vi "系统设置.vi"() -> ()   [LabVIEW 2016]
uses:
  <vilib>/Utility/miscctls.llb/LVPointTypeDef.ctl
  <vilib>/ptbypt/NI_PtbyPt.lvlib
  <vilib>/Utility/config.llb/NI_LVConfig.lvlib
  PLC/PLC.lvlib
panel:
  out "一级权限":bool
  in  "定时重启配置":bool
  in  "总磷":bool
  in  "模块启用配置":bool
  in  "短信报警设置":bool
  in  "首页显示设置":bool
  in  "跨度核查":bool
  in  "空白核查":bool
  out "选项卡控件":enum32{"自由设定", "国标协议", "流量设定"}(tab)
  in  "24H周期设置":bool[](xcontrol)
  in  "运行间隔":i16=4 min=1 max=24
  in  "流量阈值":dbl=4.0 min=1.0 max=24.0
  in  "时间阈值":u16=4 min=1 max=24
  in  "周期设置":enum16{"自由设定", "国标协议", "流量设定"}(ring)
  out "二级权限":bool
  in  "质控启动日期":string(combo)="关闭"
  in  "跨度核查时间":u16(ring)=6 items=["00H", "01H", "02H", "03H", "04H", "05H", "06H", "07H", "08H", "09H", "10H", "11H", "12H", "13H", "14H", "15H", "16H", "17H", "18H", "19H", "20H", "21H", "22H", "23H", "关闭"]
  in  "空白核查时间":u16(ring)=2 items=["00H", "01H", "02H", "03H", "04H", "05H", "06H", "07H", "08H", "09H", "10H", "11H", "12H", "13H", "14H", "15H", "16H", "17H", "18H", "19H", "20H", "21H", "22H", "23H", "关闭"]
  in  "CODCr":bool
  in  "总氮":bool
  in  "氨氮":bool
  in  "CODmn":bool
  in  "多参数":bool
  in  "输入密码":u32
  in  "布尔":bool
  in  "副屏显示设置":bool
  in  "开机启动":bool caption="氨氮禁用"
  in  "运行模式":enum16{"维护模式", "常规模式", "应急模式", "质控模式"}(ring)
  # "注：周期设置分为自由设定和国标协议两种。\n1：选择自由设定情况下：运行间隔将不可选用并变灰色，周期设置可自由手动勾选\n2：选择国标协议情况下：周期时间将由运行间隔选择的时间决定，下方周期设置被禁用并无法手动勾选。\n3：选择流量设定情况下：瞬时流量连续超过流量阈值到达时间阈值设定值，仪器将自动开启测量。"
  # "自动运行启动参数"
  # "质控频次："
  # "零点核查时间："
  # "跨度核查时间："
  # "启动周期设置"
  # "m3/S"
  # "秒"
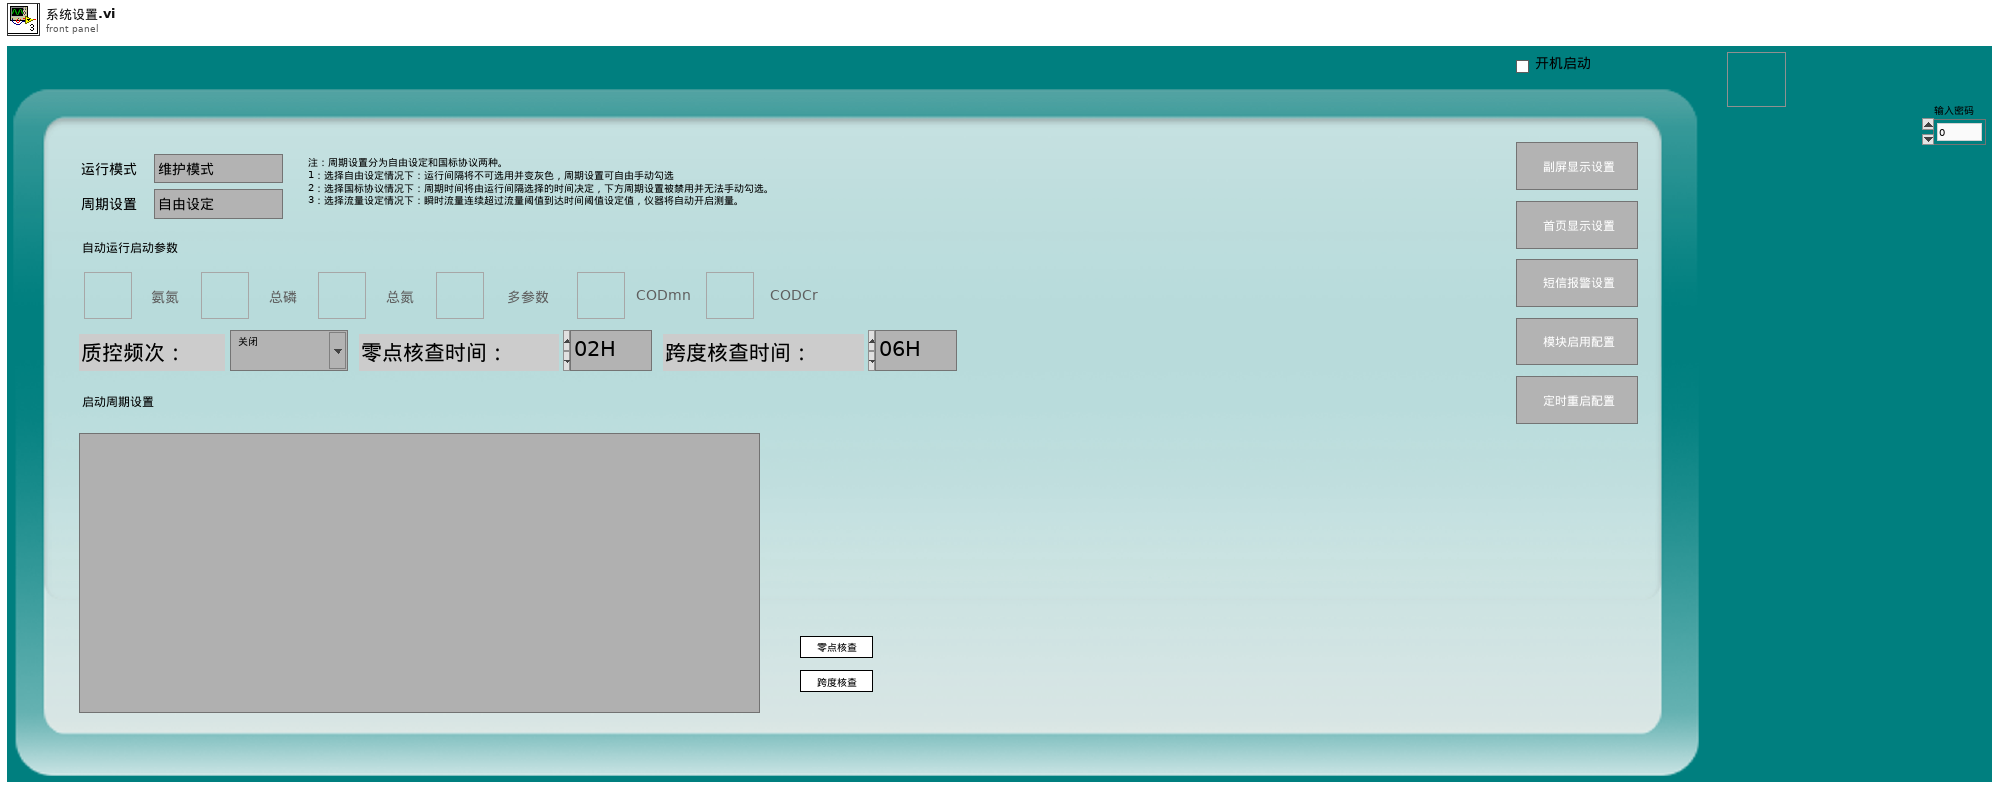
[diagram p1: front panel]
types:
  T1 = typedef "LVPointTypeDef.ctl" = cluster{"Horizontal":i16, "Vertical":i16}
  T2 = enum8{"Enabled", "Disabled", "Disabled and Grayed Out"}
  T3 = cluster{"频次":enum16{"关闭", "每天", "星期一", "星期二", "星期三", "星期四", "星期五", "星期六", "星期日"}, "时":u16, "分":u16}
  T4 = typedef "LVDateTimeRec.ctl" = cluster{"秒数的小数部分":dbl, "秒":i32, "分":i32, "时":i32, "日":i32, "月":i32, "年":i32, "天数（周）":i32, "天数（年）":i32, "DST":i32}
  T5 = enum16{"关闭", "每天", "星期一", "星期二", "星期三", "星期四", "星期五", "星期六", "星期日"}
  T6 = enum32{"Bad", "Idle", "Run top level", "Running"}
  T7 = typedef "NI_LVConfig.lvlib/Config Data RefNum.ctl" = refnum<k1>
  T8 = cluster{"运行模式":enum16{"维护模式", "常规模式", "应急模式", "质控模式"}}
  T9 = enum16{"启动测量", "标样核查", "零点核查", "跨度核查", "空白测试", "平行样测试", "加标回收", "空白校准", "标样校准", "初始化（清洗）", "停止测试", "仪器重启", "校时", "模式设置", "测量间隔设置"}
  T10 = cluster{"测量模式":enum16{"水样测量", "标样核查", "零点核查", "跨度核查", "空白测试", "加标回收", "平行样", "校零", "校标"}}
  T11 = cluster{"测试模式":enum16{"正常测试", "集成干预"}, "参数启用":cluster{"氨氮":bool, "总磷":bool, "总氮":bool, "多参数":bool, "CODMn":bool, "CODcr":bool}}
  T12 = cluster{"运行模式":enum16{"维护模式", "常规模式", "应急模式", "质控模式"}, "质控频次":enum16{"关闭", "每天", "星期一", "星期二", "星期三", "星期四", "星期五", "星期六", "星期日"}, "空白核查时间":u16, "跨度核查时间":u16, "24H周期设置":bool[]}
  T13 = enum32{"Invalid", "Standard", "Closed", "Hidden", "Minimized", "Maximized"}
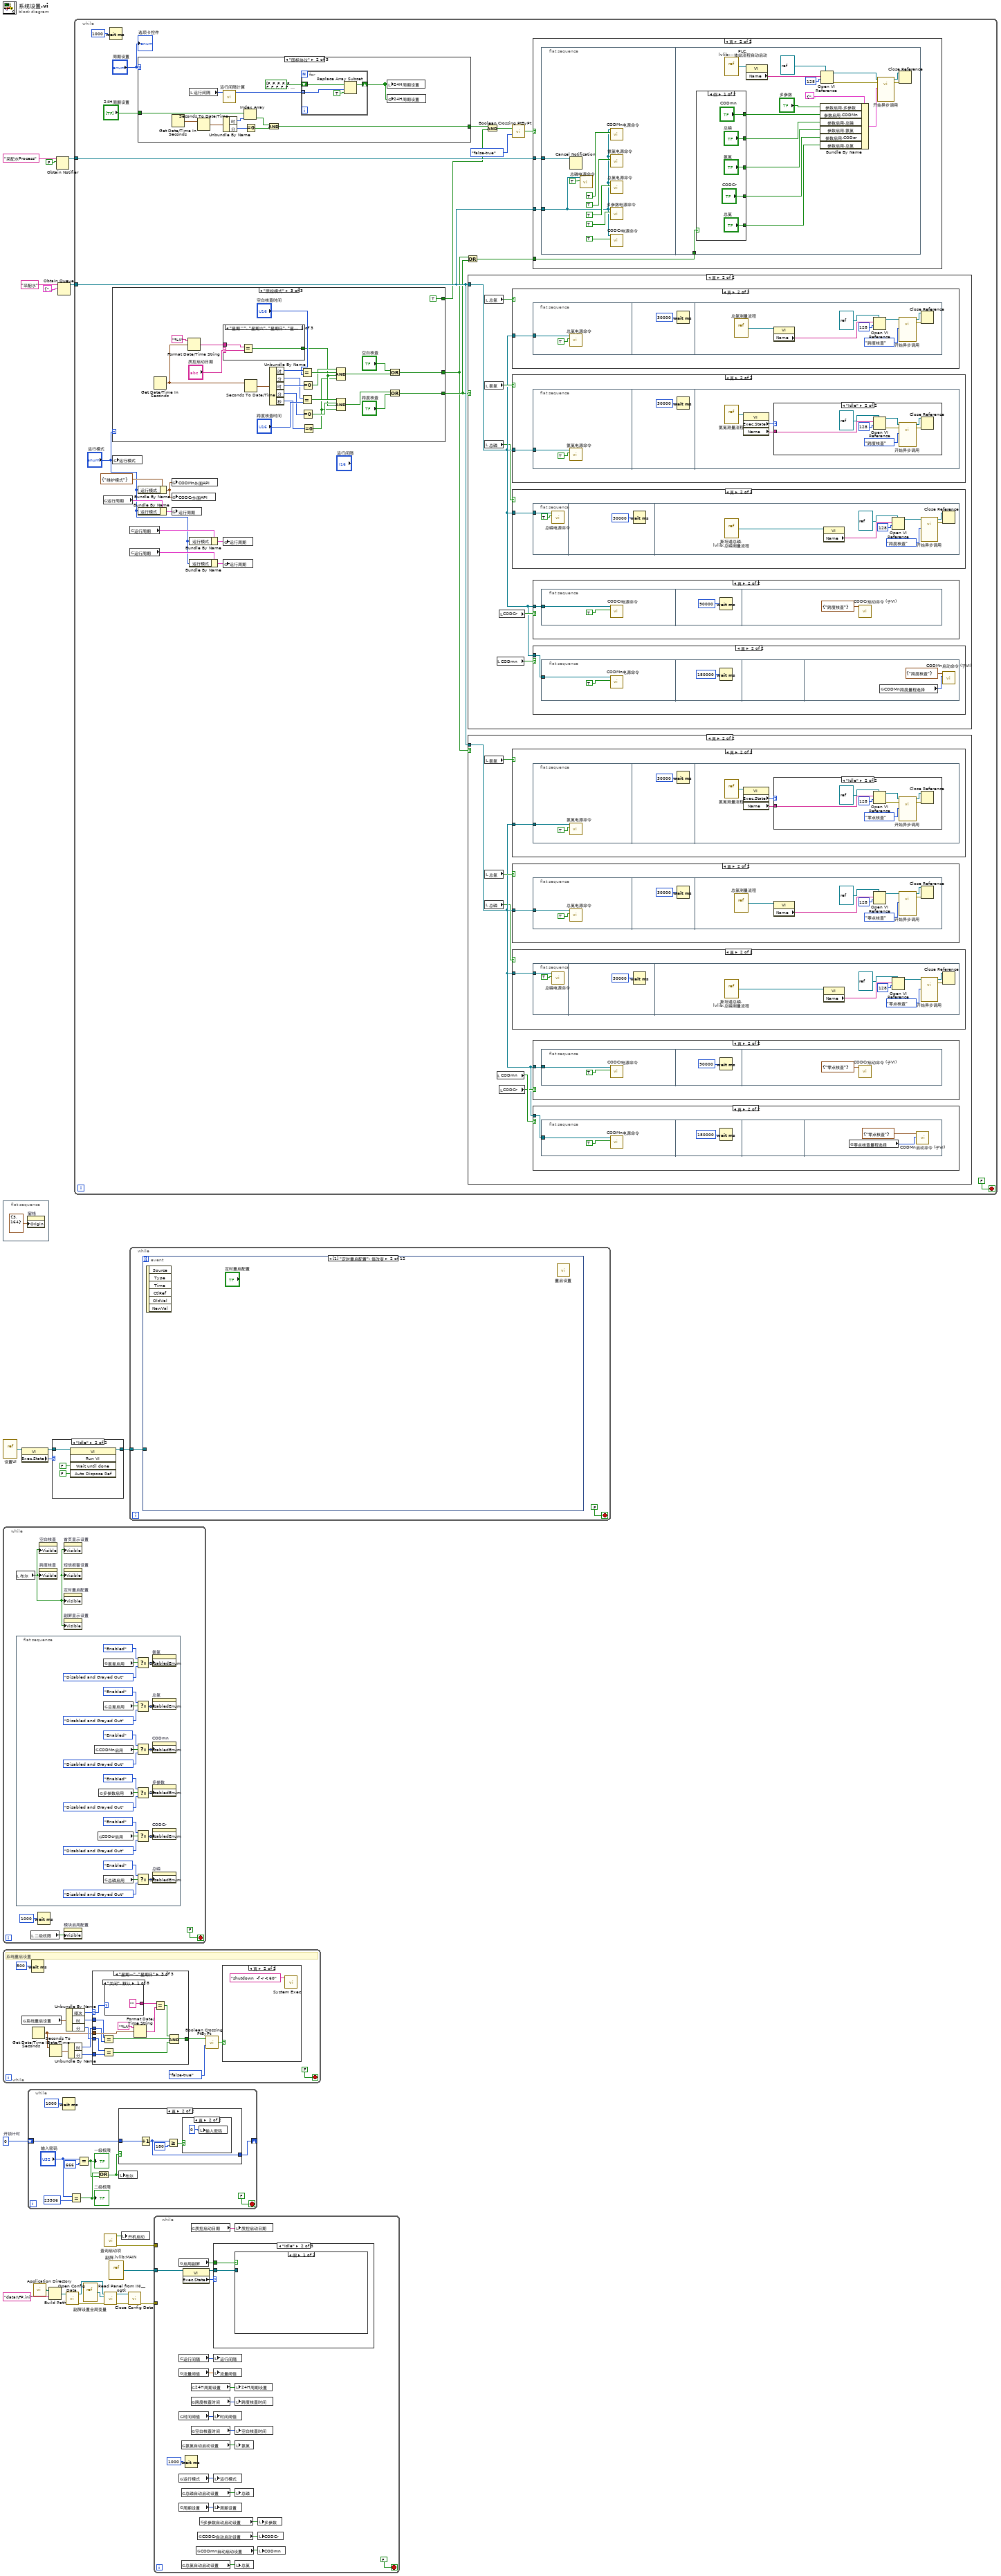
[diagram p0: block diagram]
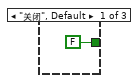
[diagram p3: hidden frame]
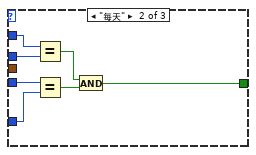
[diagram p4: hidden frame]
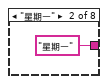
[diagram p5: hidden frame]
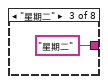
[diagram p6: hidden frame]
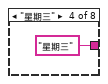
[diagram p7: hidden frame]
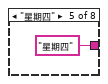
[diagram p8: hidden frame]
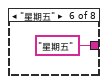
[diagram p9: hidden frame]
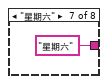
[diagram p10: hidden frame]
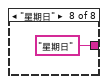
[diagram p11: hidden frame]
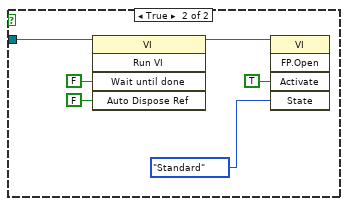
[diagram p16: hidden frame]
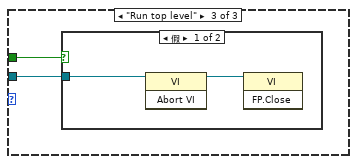
[diagram p17: hidden frame]
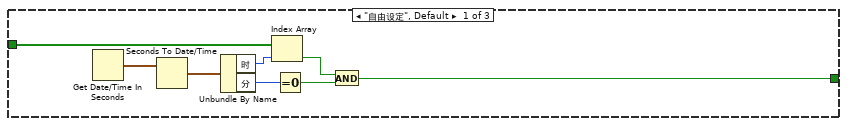
[diagram p19: hidden frame]
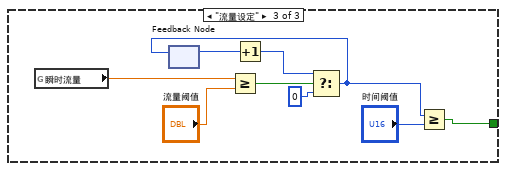
[diagram p20: hidden frame]
diagram:
  w19 = u32 0  # 开锁计时
  n1 = flat-sequence {
    frame #0 {
      n2 = property on="窗格" class="Pane"("Origin"=T1 {"Horizontal"=3, "Vertical"=164} ("原点")) -> ()  [unwired: 2 in, 2 out]
    }
  }
  n3 = vi-ref "设置UI.vi"() -> (w14:refnum<vi>)
  n4 = while {
    stop <- FALSE stop-if-true
    n5 = local read "布尔"() -> (w26:bool)
    n6 = flat-sequence {
      frame #0 {
        n7 = global read "系统设置全局变量.vi" "CODMn启用"() -> (w38:bool)
        n8 = global read "系统设置全局变量.vi" "CODcr启用"() -> (w39:bool)
        n9 = global read "系统设置全局变量.vi" "多参数启用"() -> (w37:bool)
        n10 = global read "系统设置全局变量.vi" "氨氮启用"() -> (w33:bool)
        n11 = global read "系统设置全局变量.vi" "总氮启用"() -> (w40:bool)
        n12 = global read "系统设置全局变量.vi" "总磷启用"() -> (w31:bool)
        n13 = Select(t=T2."Enabled" ("禁用"), s=w33, f=T2."Disabled and Grayed Out" ("禁用")) -> (s? t:f=w41:T2)
        n14 = Select(t=T2."Enabled" ("禁用"), s=w40, f=T2."Disabled and Grayed Out" ("禁用")) -> (s? t:f=w35:T2)
        n15 = Select(t=T2."Enabled" ("禁用"), s=w38, f=T2."Disabled and Grayed Out" ("禁用")) -> (s? t:f=w42:T2)
        n16 = Select(t=T2."Enabled" ("禁用"), s=w37, f=T2."Disabled and Grayed Out" ("禁用")) -> (s? t:f=w36:T2)
        n17 = Select(t=T2."Enabled" ("禁用"), s=w39, f=T2."Disabled and Grayed Out" ("禁用")) -> (s? t:f=w52:T2)
        n18 = Select(t=T2."Enabled" ("禁用"), s=w31, f=T2."Disabled and Grayed Out" ("禁用")) -> (s? t:f=w32:T2)
        n19 = property on="氨氮" class="Bool (严格)"("DisabledEnum"=w41) -> ()  [unwired: 2 in, 2 out]
        n20 = property on="总氮" class="Bool (严格)"("DisabledEnum"=w35) -> ()  [unwired: 2 in, 2 out]
        n21 = property on="CODmn" class="Bool (严格)"("DisabledEnum"=w42) -> ()  [unwired: 2 in, 2 out]
        n22 = property on="多参数" class="Bool (严格)"("DisabledEnum"=w36) -> ()  [unwired: 2 in, 2 out]
        n23 = property on="CODCr" class="Bool (严格)"("DisabledEnum"=w52) -> ()  [unwired: 2 in, 2 out]
        n24 = property on="总磷" class="Bool (严格)"("DisabledEnum"=w32) -> ()  [unwired: 2 in, 2 out]
      }
    }
    n25 = local read "二级权限"() -> (w25:bool)
    n26 = Wait (ms)(milliseconds to wait=u32 1000 ("等待时间（毫秒）")) -> ()  [unwired: 1 out]
    n27 = property on="空白核查" class="Bool"("Visible"=w26) -> ()  [unwired: 2 in, 2 out]
    n28 = property on="跨度核查" class="Bool"("Visible"=w26) -> ()  [unwired: 2 in, 2 out]
    n29 = property on="首页显示设置" class="Bool"("Visible"=w26) -> ()  [unwired: 2 in, 2 out]
    n30 = property on="短信报警设置" class="Bool"("Visible"=w26) -> ()  [unwired: 2 in, 2 out]
    n31 = property on="定时重启配置" class="Bool"("Visible"=w26) -> ()  [unwired: 2 in, 2 out]
    n32 = property on="副屏显示设置" class="Bool"("Visible"=w26) -> ()  [unwired: 2 in, 2 out]
    n33 = property on="模块启用配置" class="Bool"("Visible"=w25) -> ()  [unwired: 2 in, 2 out]
  }
  n34 = while {
    stop <- FALSE stop-if-true
    # "系统重启设置"
    n35 = global read "系统设置全局变量.vi" "系统重启设置"() -> (w65:T3)
    n36 = Wait (ms)(milliseconds to wait=u32 500 ("等待时间（毫秒）")) -> ()  [unwired: 1 out]
    n37 = Get Date/Time In Seconds() -> (seconds since 1Jan1904=w56:timestamp)
    n38 = Seconds To Date/Time(time stamp (now)=w56) -> (date time rec=w63:T4)  [unwired: 1 in]
    n39 = Unbundle By Name(w65) -> ("频次"=w64:T5, "时"=w60:u16, "分"=w59:u16)
    n40 = Unbundle By Name(w63) -> ("时"=w62:i32, "分"=w61:i32)
    n41 = case shown="\"星期一\"..\"星期日\"" w64 {
      selector: w64 -> [_ _ w85]
      tunnel: [FALSE w68 w75] -> w55
      tunnel: w62 -> [_ w74 w79]
      tunnel: w61 -> [_ w71 w77]
      tunnel: w60 -> [_ w73 w80]
      tunnel: w59 -> [_ w72 w78]
      tunnel: w56 -> [_ _ w86]
      frame "关闭", Default {
      }
      frame "每天" {
        n42 = Equal?(x=w73, y=w74) -> (x = y?=w69:bool)
        n43 = Equal?(x=w72, y=w71) -> (x = y?=w70:bool)
        n44 = And(x=w69, y=w70) -> (x .and. y?=w68:bool)
      }
      frame "星期一".."星期日" {
        n45 = Equal?(x=w80, y=w79) -> (x = y?=w81:bool)
        n46 = Equal?(x=w78, y=w77) -> (x = y?=w82:bool)
        n47 = case shown="\"关闭\", 默认" w85 {
          tunnel: ["" ("时间格式字符串(%c)") "星期一" ("时间格式字符串(%c)") "星期二" ("时间格式字符串(%c)") "星期三" ("时间格式字符串(%c)") "星期四" ("时间格式字符串(%c)") "星期五" ("时间格式字符串(%c)") "星期六" ("时间格式字符串(%c)") "星期日" ("时间格式字符串(%c)")] -> w83
          frame "关闭", Default {
          }
          frame "星期一" {
          }
          frame "星期二" {
          }
          frame "星期三" {
          }
          frame "星期四" {
          }
          frame "星期五" {
          }
          frame "星期六" {
          }
          frame "星期日" {
          }
        }
        n48 = Format Date/Time String(time format string (%c)="%A" ("时间格式字符串(%c)"), seconds (now)=w86) -> (date/time string=w84:string)  [unwired: 1 in]
        n49 = Equal?(x=w83, y=w84) -> (x = y?=w76:bool)
        n50 = Compound Arithmetic op=AND ("复合运算")(w76, w81, w82) -> (w75:bool)
      }
    }
    n51 = call <vilib>:"Boolean Crossing PtByPt.vi"("direction"=enum16{"either", "false-true", "true-false"}."false-true", "input"=w55) -> ("crossing"=w53:bool)  [unwired: 1 in]
    n52 = case shown="真" w53 {
      frame False {
      }
      frame True {
        n53 = call <vilib>:"System Exec.vi"("command line"="shutdown  -f -r -t 60") -> ()  [unwired: 7 in, 4 out]
      }
    }
  }
  n54 = property class="VI"(reference=w14) -> (reference out=w12:refnum<vi>, "Exec.State"=w13:T6)  [unwired: 1 in, 1 out]
  n55 = while {
    shift-right: [w101] -> _
    shift-left: w19 -> [w102]
    stop <- FALSE stop-if-true
    n56 = Wait (ms)(milliseconds to wait=u32 1000 ("等待时间（毫秒）")) -> ()  [unwired: 1 out]
    n57 = Equal?(x="输入密码", y=u32 23506) -> (x = y?=w98:bool)
    "二级权限" <- w98
    n58 = Equal?(x="输入密码", y=u32 666) -> (x = y?=w97:bool)
    "一级权限" <- w97
    n59 = Or(x=w98, y=w97) -> (x .or. y?=w96:bool)
    n60 = case shown="真" w96 {
      tunnel: w102 -> [_ w109]
      tunnel: [_ w108] -> w101
      frame False {
      }
      frame True {
        n61 = Increment(x=w109) -> (x+1=w108:u32)
        n62 = Greater Or Equal?(x=w108, y=u32 180) -> (x >= y?=w106:bool)
        n63 = case shown="真" w106 {
          frame False {
          }
          frame True {
            n64 = local write "输入密码"(u32 0 ("输入密码")) -> ()
          }
        }
      }
    }
    n65 = local write "布尔"(w96) -> ()
  }
  n66 = call <vilib>:"Application Directory.vi"() -> ("Application Directory"=w1:path)
  n67 = Build Path(base path=w1, name or relative path="data\\FP.ini" ("名称或相对路径")) -> (appended path=w8:path)
  n68 = case shown="\"Idle\"" w13 {
    tunnel: w12 -> [w111 w115]
    tunnel: [w111 w114] -> w11
    frame "Bad", Default {
    }
    frame "Idle" {
      n69 = invoke class="VI" method="Run VI"(reference=w115, "Wait until done"=FALSE ("结束前等待"), "Auto Dispose Ref"=FALSE ("自动销毁引用")) -> (reference out=w114:refnum<vi>)  [unwired: 2 in, 4 out]
    }
  }
  n70 = Obtain Notifier(name (unnamed)="采配水Process" ("名称（未命名）"), notification data type=FALSE) -> (notifier out=w21:refnum<notifier>)  [unwired: 2 in, 2 out]
  n71 = Obtain Queue(name (unnamed)="采配水" ("名称（未命名）"), element data type=cluster{"命令":string, "数据":variant} {"命令"="", "数据"=variant}) -> (queue out=w16:refnum<queue>)  [unwired: 3 in, 2 out]
  n72 = call <vilib>:"Open Config Data.vi"("configuration file path"=w8) -> ("error out"=w7:errorcluster, "refnum"=w4:T7)  [unwired: 8 in, 1 out]
  n73 = while {
    tunnel: w21 -> [w136]
    tunnel: w16 -> [w132]
    stop <- FALSE stop-if-true
    n74 = global read "氨氮断电保存全局变量.vi" "运行周期"() -> (w122:T12)
    n75 = Wait (ms)(milliseconds to wait=u32 1000 ("等待时间（毫秒）")) -> ()  [unwired: 1 out]
    n76 = case shown="\"质控模式\"" "运行模式" {
      tunnel: [_ _ w318] -> w125
      tunnel: [_ _ w322] -> w124
      tunnel: [_ TRUE TRUE] -> w129
      frame "维护模式", Default {
      }
      frame "常规模式" {
      }
      frame "质控模式" {
        n77 = Get Date/Time In Seconds() -> (seconds since 1Jan1904=w329:timestamp)
        n78 = Format Date/Time String(time format string (%c)="%A" ("时间格式字符串(%c)"), seconds (now)=w329) -> (date/time string=w327:string)  [unwired: 1 in]
        n79 = case shown="\"星期二\", \"星期六\", \"星期日\", \"星期三\", \"星期四\", \"星期五\", \"星期一\"" "质控启动日期" {
          selector: "质控启动日期" -> [w345 _ _]
          tunnel: [w344 TRUE FALSE] -> w330
          tunnel: w327 -> [w343 _ _]
          frame "星期二", "星期六", "星期日", "星期三", "星期四", "星期五", "星期一" {
            n80 = Equal?(x=w343, y=w345) -> (x = y?=w344:bool)
          }
          frame "每天" {
          }
          frame "关闭", Default {
          }
        }
        n81 = Seconds To Date/Time(time stamp (now)=w329) -> (date time rec=w342:T4)  [unwired: 1 in]
        n82 = Unbundle By Name(w342) -> ("时"=w341:i32, "分"=w339:i32, "时"=w335:i32, "分"=w334:i32, "秒"=w326:i32)
        n83 = Equal?(x=w341, y="空白核查时间") -> (x = y?=w338:bool)
        n84 = Equal?(x=w335, y="跨度核查时间") -> (x = y?=w333:bool)
        n85 = Equal To 0?(x=w339) -> (x = 0?=w337:bool)
        n86 = Equal To 0?(x=w334) -> (x = 0?=w332:bool)
        n87 = Equal To 0?(x=w326) -> (x = 0?=w325:bool)
        n88 = Compound Arithmetic op=AND ("复合运算")(w337, w338, w330, w325) -> (w323:bool)
        n89 = Compound Arithmetic op=AND ("复合运算")(w333, w332, w330, w325) -> (w320:bool)
        n90 = Or(x="空白核查", y=w323) -> (x .or. y?=w322:bool)
        n91 = Or(x=w320, y="跨度核查") -> (x .or. y?=w318:bool)
      }
    }
    n92 = global write "多参数全局变量.vi" "运行模式"("运行模式") -> ()
    n93 = global read "总氮断电保存全局变量.vi" "运行周期"() -> (w120:T12)
    n94 = global read "总磷断电保存全局变量.vi" "运行周期"() -> (w118:T12)
    n95 = case shown="\"国标协议\"" "周期设置" {
      tunnel: [w140 w147 w163] -> w128
      tunnel: "24H周期设置" -> [w139 w148 _]
      frame "自由设定", Default {
        n96 = Get Date/Time In Seconds() -> (seconds since 1Jan1904=w141:timestamp)
        n97 = Seconds To Date/Time(time stamp (now)=w141) -> (date time rec=w142:T4)  [unwired: 1 in]
        n98 = Unbundle By Name(w142) -> ("时"=w145:i32, "分"=w143:i32)
        n99 = Index Array(array=w139, index=w145) -> (element=w146:bool)
        n100 = Equal To 0?(x=w143) -> (x = 0?=w144:bool)
        n101 = And(x=w146, y=w144) -> (x .and. y?=w140:bool)
      }
      frame "国标协议" {
        n102 = Get Date/Time In Seconds() -> (seconds since 1Jan1904=w149:timestamp)
        n103 = local read "运行间隔"() -> (w158:i16)
        n104 = Seconds To Date/Time(time stamp (now)=w149) -> (date time rec=w150:T4)  [unwired: 1 in]
        n105 = call "运行间隔计算.vi"("运行周期"=w158) -> ("数组"=w157:i32[])  [unwired: 10 in]
        n106 = Unbundle By Name(w150) -> ("时"=w153:i32, "分"=w151:i32)
        n107 = Index Array(array=w148, index=w153) -> (element=w154:bool)
        n108 = Equal To 0?(x=w151) -> (x = 0?=w152:bool)
        n109 = And(x=w154, y=w152) -> (x .and. y?=w147:bool)
        n110 = for {
          tunnel: w157 -> [w161] mode=indexing
          shift-right: [w159] -> w155
          shift-left: bool[] [FALSE, FALSE, FALSE, FALSE, FALSE, FALSE, FALSE, FALSE, FALSE, FALSE, FALSE, FALSE, FALSE, FALSE, FALSE, FALSE, FALSE, FALSE, FALSE, FALSE, FALSE, FALSE, FALSE, FALSE] ("24H周期设置") -> [w162]
          n111 = Replace Array Subset(array=w162, new element=TRUE ("新元素/子数组"), index=w161) -> (w159:bool[])
        }
        n112 = local write "24H周期设置"(w155) -> ()
        n113 = global write "系统设置全局变量.vi" "24H周期设置"(w155) -> ()
      }
      frame "流量设定" {
        n114 = global read "流量计全局变量.vi" "瞬时流量"() -> (w171:dbl)
        n115 = feedback #1() -> (w168:i16)  [unwired: 1 in]
        n116 = Greater Or Equal?(x=w171, y="流量阈值") -> (x >= y?=w166:bool)
        n117 = Increment(x=w168) -> (x+1=w167:i16)
        n118 = Select(t=w167, s=w166, f=i16 0) -> (s? t:f=w165:i16)
        n119 = feedback-in #1(w165) -> ()
        n120 = Greater Or Equal?(x=w165, y="时间阈值") -> (x >= y?=w163:bool)
      }
    }
    n121 = Bundle By Name(cluster=T8 {"运行模式"=enum."维护模式"} ("外围API"), "运行模式"="运行模式") -> (w126:T8)
    n122 = Bundle By Name(cluster=w122, "运行模式"="运行模式") -> (w121:T12)
    n123 = global write "CODMN外部API.vi" "CODMn外围API"(w126) -> ()
    n124 = global write "CODCr外部API.vi" "CODCr外围API"(w126) -> ()
    n125 = global write "氨氮断电保存全局变量.vi" "运行周期"(w121) -> ()
    n126 = Bundle By Name(cluster=w120, "运行模式"="运行模式") -> (w119:T12)
    n127 = Bundle By Name(cluster=w118, "运行模式"="运行模式") -> (w117:T12)
    n128 = global write "总氮断电保存全局变量.vi" "运行周期"(w119) -> ()
    n129 = global write "总磷断电保存全局变量.vi" "运行周期"(w117) -> ()
    n130 = Or(x=w124, y=w125) -> (x .or. y?=w123:bool)
    n131 = case shown="真" w125 {
      tunnel: w132 -> [_ w173]
      frame False {
      }
      frame True {
        n132 = local read "总氮"() -> (w176:bool)
        n133 = local read "氨氮"() -> (w177:bool)
        n134 = local read "总磷"() -> (w172:bool)
        n135 = local read "CODmn"() -> (w175:bool)
        n136 = local read "CODCr"() -> (w174:bool)
        n137 = case shown="真" w176 {
          tunnel: w173 -> [_ w201]
          frame False {
          }
          frame True {
            n138 = flat-sequence {
              tunnel: w201 -> [w203]
              frame #0 {
                n139 = call "总氮电源命令.vi"("通电/断电"=TRUE, "队列"=w203) -> ()  [unwired: 9 in, 1 out]
              }
              frame #1 {
                n140 = Wait (ms)(milliseconds to wait=u32 30000 ("等待时间（毫秒）")) -> ()  [unwired: 1 out]
              }
              frame #2 {
                n141 = vi-ref "总氮测量流程.vi"() -> (w210:refnum<vi>)
                n142 = property class="VI"(reference=w210) -> ("Name"=w211:string)  [unwired: 1 in, 2 out]
                n143 = Open VI Reference(type specifier VI Refnum (for type only)=refnum<vi> refnum, vi path=w211, options=128 ("选项")) -> (vi reference=w209:refnum<vi>)  [unwired: 3 in, 1 out]
                n144 = call-by-ref "开始异步调用"(reference=w209, "控制命令"=T9."跨度核查") -> (reference out=w208:refnum<vi>, error out=w207:errorcluster)  [unwired: 12 in]
                n145 = Close Reference(reference=w208, error in (no error)=w207) -> ()  [unwired: 1 out]
              }
            }
          }
        }
        n146 = case shown="真" w177 {
          tunnel: w173 -> [_ w213]
          frame False {
          }
          frame True {
            n147 = flat-sequence {
              tunnel: w213 -> [w214]
              frame #0 {
                n148 = call "氨氮电源命令.vi"("通电/断电"=TRUE, "队列"=w214) -> ()  [unwired: 9 in, 1 out]
              }
              frame #1 {
                n149 = Wait (ms)(milliseconds to wait=u32 30000 ("等待时间（毫秒）")) -> ()  [unwired: 1 out]
              }
              frame #2 {
                n150 = vi-ref "氨氮测量流程.vi"() -> (w219:refnum<vi>)
                n151 = property class="VI"(reference=w219) -> ("Exec.State"=w217:T6, "Name"=w218:string)  [unwired: 1 in, 2 out]
                n152 = case shown="\"Idle\"" w217 {
                  tunnel: w218 -> [_ w224]
                  frame "Bad", Default {
                  }
                  frame "Idle" {
                    n153 = Open VI Reference(type specifier VI Refnum (for type only)=refnum<vi> refnum, vi path=w224, options=128 ("选项")) -> (vi reference=w222:refnum<vi>, error out=w225:errorcluster)  [unwired: 3 in]
                    n154 = call-by-ref "开始异步调用"(reference=w222, error in=w225, "控制命令"=T9."跨度核查") -> (reference out=w226:refnum<vi>, error out=w227:errorcluster)  [unwired: 11 in]
                    n155 = Close Reference(reference=w226, error in (no error)=w227) -> ()  [unwired: 1 out]
                  }
                }
              }
            }
          }
        }
        n156 = case shown="真" w172 {
          tunnel: w173 -> [_ w178]
          frame False {
          }
          frame True {
            n157 = flat-sequence {
              tunnel: w178 -> [w180]
              frame #0 {
                n158 = call "总磷电源命令.vi"("通电/断电"=TRUE, "队列"=w180) -> ()  [unwired: 9 in, 1 out]
              }
              frame #1 {
                n159 = Wait (ms)(milliseconds to wait=u32 30000 ("等待时间（毫秒）")) -> ()  [unwired: 1 out]
              }
              frame #2 {
                n160 = vi-ref "斯坦道总磷.lvlib:总磷测量流程.vi"() -> (w187:refnum<vi>)
                n161 = property class="VI"(reference=w187) -> ("Name"=w188:string)  [unwired: 1 in, 2 out]
                n162 = Open VI Reference(type specifier VI Refnum (for type only)=refnum<vi> refnum, vi path=w188, options=128 ("选项")) -> (vi reference=w186:refnum<vi>)  [unwired: 3 in, 1 out]
                n163 = call-by-ref "开始异步调用"(reference=w186, "控制命令"=T9."跨度核查") -> (reference out=w185:refnum<vi>, error out=w184:errorcluster)  [unwired: 12 in]
                n164 = Close Reference(reference=w185, error in (no error)=w184) -> ()  [unwired: 1 out]
              }
            }
          }
        }
        n165 = case shown="真" w174 {
          tunnel: w173 -> [_ w190]
          frame False {
          }
          frame True {
            n166 = flat-sequence {
              tunnel: w190 -> [w191]
              frame #0 {
                n167 = call "CODCr电源命令.vi"("通电/断电"=TRUE, "队列"=w191) -> ()  [unwired: 9 in, 1 out]
              }
              frame #1 {
                n168 = Wait (ms)(milliseconds to wait=u32 90000 ("等待时间（毫秒）")) -> ()  [unwired: 1 out]
              }
              frame #2 {
                n169 = call "CODCr启动命令 (子VI).vi"("启动测量模式"=T10 {"测量模式"=enum."跨度核查"}) -> ()  [unwired: 11 in]
              }
            }
          }
        }
        n170 = case shown="真" w175 {
          tunnel: w173 -> [_ w195]
          frame False {
          }
          frame True {
            n171 = flat-sequence {
              tunnel: w195 -> [w196]
              frame #0 {
                n172 = call "CODMn电源命令.vi"("通电/断电"=TRUE, "队列"=w196) -> ()  [unwired: 9 in, 1 out]
              }
              frame #1 {
                n173 = Wait (ms)(milliseconds to wait=u32 180000 ("等待时间（毫秒）")) -> ()  [unwired: 1 out]
              }
              frame #2 {
              }
              frame #3 {
                n174 = global read "CODMn断电保存全局变量.vi" "CODMn跨度量程选择"() -> (w199:enum32{"H", "L", "AUTO"})
                n175 = call "CODMn启动命令 (子VI).vi"("CODMn量程切换"=w199, "启动测量模式"=T10 {"测量模式"=enum."跨度核查"}) -> ()  [unwired: 10 in]
              }
            }
          }
        }
      }
    }
    n176 = case shown="真" w124 {
      tunnel: w132 -> [_ w229]
      frame False {
      }
      frame True {
        n177 = local read "氨氮"() -> (w233:bool)
        n178 = local read "总氮"() -> (w232:bool)
        n179 = local read "总磷"() -> (w228:bool)
        n180 = local read "CODmn"() -> (w231:bool)
        n181 = local read "CODCr"() -> (w230:bool)
        n182 = case shown="真" w233 {
          tunnel: w229 -> [_ w269]
          frame False {
          }
          frame True {
            n183 = flat-sequence {
              tunnel: w269 -> [w270]
              frame #0 {
                n184 = call "氨氮电源命令.vi"("通电/断电"=TRUE, "队列"=w270) -> ()  [unwired: 9 in, 1 out]
              }
              frame #1 {
                n185 = Wait (ms)(milliseconds to wait=u32 30000 ("等待时间（毫秒）")) -> ()  [unwired: 1 out]
              }
              frame #2 {
                n186 = vi-ref "氨氮测量流程.vi"() -> (w275:refnum<vi>)
                n187 = property class="VI"(reference=w275) -> ("Exec.State"=w273:T6, "Name"=w274:string)  [unwired: 1 in, 2 out]
                n188 = case shown="\"Idle\"" w273 {
                  tunnel: w274 -> [_ w280]
                  frame "Bad", Default {
                  }
                  frame "Idle" {
                    n189 = Open VI Reference(type specifier VI Refnum (for type only)=refnum<vi> refnum, vi path=w280, options=128 ("选项")) -> (vi reference=w278:refnum<vi>, error out=w281:errorcluster)  [unwired: 3 in]
                    n190 = call-by-ref "开始异步调用"(reference=w278, error in=w281, "控制命令"=T9."零点核查") -> (reference out=w282:refnum<vi>, error out=w283:errorcluster)  [unwired: 11 in]
                    n191 = Close Reference(reference=w282, error in (no error)=w283) -> ()  [unwired: 1 out]
                  }
                }
              }
            }
          }
        }
        n192 = case shown="真" w232 {
          tunnel: w229 -> [_ w257]
          frame False {
          }
          frame True {
            n193 = flat-sequence {
              tunnel: w257 -> [w259]
              frame #0 {
                n194 = call "总氮电源命令.vi"("通电/断电"=TRUE, "队列"=w259) -> ()  [unwired: 9 in, 1 out]
              }
              frame #1 {
                n195 = Wait (ms)(milliseconds to wait=u32 30000 ("等待时间（毫秒）")) -> ()  [unwired: 1 out]
              }
              frame #2 {
                n196 = vi-ref "总氮测量流程.vi"() -> (w266:refnum<vi>)
                n197 = property class="VI"(reference=w266) -> ("Name"=w267:string)  [unwired: 1 in, 2 out]
                n198 = Open VI Reference(type specifier VI Refnum (for type only)=refnum<vi> refnum, vi path=w267, options=128 ("选项")) -> (vi reference=w265:refnum<vi>)  [unwired: 3 in, 1 out]
                n199 = call-by-ref "开始异步调用"(reference=w265, "控制命令"=T9."零点核查") -> (reference out=w264:refnum<vi>, error out=w263:errorcluster)  [unwired: 12 in]
                n200 = Close Reference(reference=w264, error in (no error)=w263) -> ()  [unwired: 1 out]
              }
            }
          }
        }
        n201 = case shown="真" w228 {
          tunnel: w229 -> [_ w234]
          frame False {
          }
          frame True {
            n202 = flat-sequence {
              tunnel: w234 -> [w236]
              frame #0 {
                n203 = call "总磷电源命令.vi"("通电/断电"=TRUE, "队列"=w236) -> ()  [unwired: 9 in, 1 out]
              }
              frame #1 {
                n204 = Wait (ms)(milliseconds to wait=u32 30000 ("等待时间（毫秒）")) -> ()  [unwired: 1 out]
              }
              frame #2 {
                n205 = vi-ref "斯坦道总磷.lvlib:总磷测量流程.vi"() -> (w243:refnum<vi>)
                n206 = property class="VI"(reference=w243) -> ("Name"=w244:string)  [unwired: 1 in, 2 out]
                n207 = Open VI Reference(type specifier VI Refnum (for type only)=refnum<vi> refnum, vi path=w244, options=128 ("选项")) -> (vi reference=w242:refnum<vi>)  [unwired: 3 in, 1 out]
                n208 = call-by-ref "开始异步调用"(reference=w242, "控制命令"=T9."零点核查") -> (reference out=w241:refnum<vi>, error out=w240:errorcluster)  [unwired: 12 in]
                n209 = Close Reference(reference=w241, error in (no error)=w240) -> ()  [unwired: 1 out]
              }
            }
          }
        }
        n210 = case shown="真" w230 {
          tunnel: w229 -> [_ w246]
          frame False {
          }
          frame True {
            n211 = flat-sequence {
              tunnel: w246 -> [w247]
              frame #0 {
                n212 = call "CODCr电源命令.vi"("通电/断电"=TRUE, "队列"=w247) -> ()  [unwired: 9 in, 1 out]
              }
              frame #1 {
                n213 = Wait (ms)(milliseconds to wait=u32 90000 ("等待时间（毫秒）")) -> ()  [unwired: 1 out]
              }
              frame #2 {
                n214 = call "CODCr启动命令 (子VI).vi"("启动测量模式"=T10 {"测量模式"=enum."零点核查"}) -> ()  [unwired: 11 in]
              }
            }
          }
        }
        n215 = case shown="真" w231 {
          tunnel: w229 -> [_ w251]
          frame False {
          }
          frame True {
            n216 = flat-sequence {
              tunnel: w251 -> [w252]
              frame #0 {
                n217 = call "CODMn电源命令.vi"("通电/断电"=TRUE, "队列"=w252) -> ()  [unwired: 9 in, 1 out]
              }
              frame #1 {
                n218 = Wait (ms)(milliseconds to wait=u32 180000 ("等待时间（毫秒）")) -> ()  [unwired: 1 out]
              }
              frame #2 {
              }
              frame #3 {
                n219 = global read "CODMn断电保存全局变量.vi" "零点核查量程选择"() -> (w255:enum32{"H", "L", "AUTO"})
                n220 = call "CODMn启动命令 (子VI).vi"("CODMn量程切换"=w255, "启动测量模式"=T10 {"测量模式"=enum."零点核查"}) -> ()  [unwired: 10 in]
              }
            }
          }
        }
      }
    }
    n221 = And(x=w128, y=w129) -> (x .and. y?=w127:bool)
    n222 = call <vilib>:"Boolean Crossing PtByPt.vi"("direction"=enum16{"either", "false-true", "true-false"}."false-true", "input"=w127) -> ("crossing"=w134:bool)  [unwired: 1 in]
    n223 = case shown="真" w134 {
      tunnel: w136 -> [_ w286]
      tunnel: w132 -> [_ w285]
      tunnel: w123 -> [_ w284]
      frame False {
      }
      frame True {
        n224 = flat-sequence {
          tunnel: w286 -> [w294]
          tunnel: w285 -> [w288]
          tunnel: w284 -> [w300]
          frame #0 {
            n225 = Cancel Notification(0:w294) -> ()  [unwired: 1 in, 3 out]
            n226 = call "总磷电源命令.vi"("通电/断电"=TRUE, "队列"=w288) -> ()  [unwired: 9 in, 1 out]
            n227 = call "CODMn电源命令.vi"("通电/断电"=TRUE, "队列"=w288) -> ()  [unwired: 9 in, 1 out]
            n228 = call "氨氮电源命令.vi"("通电/断电"=TRUE, "队列"=w288) -> ()  [unwired: 9 in, 1 out]
            n229 = call "总氮电源命令.vi"("通电/断电"=TRUE, "队列"=w288) -> ()  [unwired: 9 in, 1 out]
            n230 = call "多参数电源命令.vi"("通电/断电"=TRUE, "队列"=w288) -> ()  [unwired: 9 in, 1 out]
            n231 = call "CODCr电源命令.vi"("通电/断电"=TRUE, "队列"=w288) -> ()  [unwired: 9 in, 1 out]
          }
          frame #1 {
            n232 = case shown="假" w300 {
              tunnel: ["CODmn" _] -> w310
              tunnel: ["总氮" _] -> w296
              tunnel: ["CODCr" _] -> w309
              tunnel: ["氨氮" _] -> w308
              tunnel: ["总磷" _] -> w295
              frame False {
              }
              frame True {
              }
            }
            n233 = vi-ref "PLC.lvlib:一体站流程自动启动.vi"() -> (w305:refnum<vi>)
            n234 = property class="VI"(reference=w305) -> ("Name"=w306:string)  [unwired: 1 in, 2 out]
            n235 = Bundle By Name(cluster=T11 {"测试模式"=enum."正常测试", "参数启用"={"氨氮"=FALSE, "总磷"=FALSE, "总氮"=FALSE, "多参数"=FALSE, "CODMn"=FALSE, "CODcr"=FALSE}} ("参数"), "参数启用.多参数"="多参数", "参数启用.CODMn"=w310, "参数启用.总磷"=w295, "参数启用.氨氮"=w308, "参数启用.CODcr"=w309, "参数启用.总氮"=w296) -> (w297:T11)
            n236 = Open VI Reference(type specifier VI Refnum (for type only)=refnum<vi> refnum, vi path=w306, options=128 ("选项")) -> (vi reference=w304:refnum<vi>, error out=w303:errorcluster)  [unwired: 3 in]
            n237 = call-by-ref "开始异步调用"(reference=w304, error in=w303, "参数"=w297) -> (reference out=w302:refnum<vi>, error out=w301:errorcluster)  [unwired: 11 in]
            n238 = Close Reference(reference=w302, error in (no error)=w301) -> ()  [unwired: 1 out]
          }
        }
      }
    }
    "选项卡控件" <- "周期设置"
  }
  n239 = vi-ref "副屏设置全局变量.vi"() -> (w5:refnum<vi>)
  n240 = call "查询启动项.vi"() -> ("error out"=w10:errorcluster, "包含启动项"=w20:bool)  [unwired: 10 in]
  n241 = call <userlib>:"Read Panel from INI__ogtk.vi"("error in (no error)"=w7, "VI ref"=w5, "refnum"=w4) -> ("error out"=w6:errorcluster, "refnum out"=w3:T7)  [unwired: 7 in]
  n242 = vi-ref "副屏.lvlib:MAIN.vi"() -> (w15:refnum<vi>)
  n243 = local write "开机启动"(w20) -> ()
  n244 = call <vilib>:"Close Config Data.vi"("error in (no error)"=w6, "refnum"=w3) -> ("error out"=w2:errorcluster)  [unwired: 8 in, 1 out]
  n245 = while {
    tunnel: w11 -> [w348]
    stop <- FALSE stop-if-true
    n246 = event shown="[1] \"定时重启配置\": 值改变" {
      selector: _ -> [_ _ _ _ _ _ _ _ _ _ _ _]
      dyn-events: _ -> [_ _ _ _ _ _ _ _ _ _ _ _]
      timeout: _ -> [_ _ _ _ _ _ _ _ _ _ _ _]
      tunnel: w348 -> [_ _ _ _ _ _ _ _ _ _ w402 _]
      event Timeout {
        n247 = event-data() -> ()  [unwired: 1 in, 3 out]
      }
      event "定时重启配置": Value Change {
        n248 = event-data() -> ()  [unwired: 1 in, 6 out]
        n249 = call "重启设置.vi"() -> ()  [unwired: 12 in]
      }
      event "模块启用配置": Value Change {
        n250 = event-data() -> ()  [unwired: 1 in, 6 out]
        n251 = call "模块启用配置框.vi"() -> ()  [unwired: 12 in]
      }
      event "24H周期设置", "运行模式", "多参数", "CODmn", "氨氮", "总氮", "CODCr", "质控启动日期", "空白核查时间", "跨度核查时间", "运行间隔", "周期设置", "流量阈值", "时间阈值", "总磷": Value Change {
        n252 = event-data() -> ()  [unwired: 1 in, 6 out]
        n253 = flat-sequence {
          frame #0 {
            n254 = local read "氨氮"() -> (w363:bool)
            n255 = local read "总氮"() -> (w361:bool)
            n256 = local read "总磷"() -> (w350:bool)
            n257 = local read "运行间隔"() -> (w354:i16)
            n258 = local read "周期设置"() -> (w353:enum16{"自由设定", "国标协议", "流量设定"})
            n259 = local read "流量阈值"() -> (w351:dbl)
            n260 = local read "时间阈值"() -> (w352:u16)
            n261 = local read "运行模式"() -> (w364:enum16{"维护模式", "常规模式", "应急模式", "质控模式"})
            n262 = local read "CODmn"() -> (w360:bool)
            n263 = local read "CODCr"() -> (w362:bool)
            n264 = local read "多参数"() -> (w359:bool)
            n265 = local read "24H周期设置"() -> (w358:bool[])
            n266 = local read "空白核查时间"() -> (w356:u16)
            n267 = local read "质控启动日期"() -> (w357:string)
            n268 = local read "跨度核查时间"() -> (w355:u16)
            n269 = global write "系统设置全局变量.vi" "氨氮自动启动设置"(w363) -> ()
            n270 = global write "系统设置全局变量.vi" "总氮自动启动设置"(w361) -> ()
            n271 = global write "系统设置全局变量.vi" "总磷自动启动设置"(w350) -> ()
            n272 = global write "系统设置全局变量.vi" "运行间隔"(w354) -> ()
            n273 = global write "系统设置全局变量.vi" "周期设置"(w353) -> ()
            n274 = global write "系统设置全局变量.vi" "流量阈值"(w351) -> ()
            n275 = global write "系统设置全局变量.vi" "CODCr自动启动设置"(w362) -> ()
            n276 = global write "系统设置全局变量.vi" "CODmn自动启动设置"(w360) -> ()
            n277 = global write "系统设置全局变量.vi" "时间阈值"(w352) -> ()
            n278 = global write "系统设置全局变量.vi" "多参数自动启动设置"(w359) -> ()
            n279 = global write "系统设置全局变量.vi" "运行模式"(w364) -> ()
            n280 = global write "系统设置全局变量.vi" "24H周期设置"(w358) -> ()
            n281 = global write "系统设置全局变量.vi" "空白核查时间"(w356) -> ()
            n282 = global write "系统设置全局变量.vi" "质控启动日期"(w357) -> ()
            n283 = global write "系统设置全局变量.vi" "跨度核查时间"(w355) -> ()
          }
          frame #1 {
            n284 = call <vilib>:"Application Directory.vi"() -> ("Application Directory"=w378:path)
            n285 = Build Path(base path=w378, name or relative path="data\\sys.ini" ("名称或相对路径")) -> (appended path=w376:path)
            n286 = call <vilib>:"Open Config Data.vi"("configuration file path"=w376) -> ("error out"=w372:errorcluster, "refnum"=w375:T7)  [unwired: 8 in, 1 out]
            n287 = vi-ref "系统设置全局变量.vi"() -> (w374:refnum<vi>)
            n288 = call <userlib>:"Write Panel to INI__ogtk.vi"("error in (no error)"=w372, "VI ref"=w374, "refnum"=w375) -> ("error out"=w371:errorcluster, "refnum out"=w373:T7)  [unwired: 7 in]
            n289 = call <vilib>:"Close Config Data.vi"("error in (no error)"=w371, "refnum"=w373) -> ("error out"=w366:errorcluster, "file path"=w365:path)  [unwired: 8 in]
            n290 = Open/Create/Replace File(file path (use dialog)=w365, error in=w366) -> (refnum out=w369:refnum<file>, error out=w370:errorcluster)  [unwired: 4 in, 1 out]
            n291 = Flush File(refnum=w369, error in=w370) -> (refnum out=w368:refnum<file>, error out=w367:errorcluster)
            n292 = Close File(refnum=w368, error in=w367) -> ()  [unwired: 2 out]
          }
        }
      }
      event "运行间隔": Mouse Down {
        n293 = event-data() -> ("CtlRef"=w382:refnum<vi>)  [unwired: 1 in, 7 out]
        n294 = property class="DigNum (严格)"(reference=w382) -> (reference out=w381:refnum<vi>, "Value"=w380:i16)  [unwired: 1 in, 1 out]
        n295 = call "数字键盘.vi"("OldNumber"=w380) -> ("NewNumber"=w379:sgl)
        n296 = property class="DigNum (严格)"(reference=w381, "Val(Sgnl)"=w379) -> ()  [unwired: 1 in, 2 out]
      }
      event "流量阈值": Mouse Down {
        n297 = event-data() -> ("CtlRef"=w386:refnum<vi>)  [unwired: 1 in, 7 out]
        n298 = property class="DigNum (严格)"(reference=w386) -> (reference out=w385:refnum<vi>, "Value"=w384:dbl)  [unwired: 1 in, 1 out]
        n299 = call "数字键盘.vi"("OldNumber"=w384) -> ("NewNumber"=w383:sgl)
        n300 = property class="DigNum (严格)"(reference=w385, "Val(Sgnl)"=w383) -> ()  [unwired: 1 in, 2 out]
      }
      event "时间阈值": Mouse Down {
        n301 = event-data() -> ("CtlRef"=w390:refnum<vi>)  [unwired: 1 in, 7 out]
        n302 = property class="DigNum (严格)"(reference=w390) -> (reference out=w389:refnum<vi>, "Value"=w388:u16)  [unwired: 1 in, 1 out]
        n303 = call "数字键盘.vi"("OldNumber"=w388) -> ("NewNumber"=w387:sgl)
        n304 = property class="DigNum (严格)"(reference=w389, "Val(Sgnl)"=w387) -> ()  [unwired: 1 in, 2 out]
      }
      event "开机启动": Value Change {
        n305 = event-data() -> ("NewVal"=w392:bool)  [unwired: 1 in, 5 out]
        n306 = call <vilib>:"Application Directory.vi"() -> ("Application Directory"=w391:path)
        n307 = case shown="假" w392 {
          tunnel: w391 -> [_ w397]
          frame False {
            n308 = call "删除启动项.vi"() -> ("删除标记"=w393:bool)  [unwired: 10 in, 1 out]
            n309 = case shown="真" w393 {
              frame False {
                n310 = local write "开机启动"(TRUE ("开机启动")) -> ()
                n311 = One Button Dialog(message="启动项删除失败" ("消息")) -> ()  [unwired: 1 in, 1 out]
              }
              frame True {
              }
            }
          }
          frame True {
            n312 = call "添加启动项.vi"("启动文件路径"=w397) -> ("添加成功标记"=w396:bool)  [unwired: 9 in, 1 out]
            n313 = case shown="真" w396 {
              frame False {
                n314 = local write "开机启动"(FALSE ("开机启动")) -> ()
                n315 = One Button Dialog(message="启动项添加失败" ("消息")) -> ()  [unwired: 1 in, 1 out]
              }
              frame True {
              }
            }
          }
        }
      }
      event "副屏显示设置": Value Change {
        n316 = event-data() -> ()  [unwired: 1 in, 6 out]
        n317 = call "副屏设置.vi"() -> ()  [unwired: 12 in]
      }
      event "首页显示设置": Value Change {
        n318 = event-data() -> ()  [unwired: 1 in, 6 out]
        n319 = call "首页显示设置.vi"() -> ()  [unwired: 12 in]
      }
      event "短信报警设置": Value Change {
        n320 = event-data() -> ()  [unwired: 1 in, 6 out]
        n321 = invoke class="VI" method="FP.Open"(reference=w402, "Activate"=TRUE ("激活？"), "State"=T13."Standard" ("状态")) -> ()  [unwired: 2 in, 5 out]
      }
      event "布尔": Value Change {
        n322 = event-data() -> ("OldVal"=w404:bool)  [unwired: 1 in, 5 out]
        n323 = case shown="假" w404 {
          tunnel: [w405 _] -> w403
          frame False {
            n324 = call "数字密码键盘.vi"() -> ("NewNumber"=w405:sgl)  [unwired: 1 in]
          }
          frame True {
          }
        }
        n325 = local write "输入密码"(w403) -> ()
      }
    }
  }
  n326 = while {
    tunnel: w15 -> [w418]
    tunnel: w10 -> [_]
    tunnel: w2 -> [_]
    stop <- FALSE stop-if-true
    n327 = global read "副屏设置全局变量.vi" "启用副屏"() -> (w416:bool)
    n328 = global read "系统设置全局变量.vi" "运行间隔"() -> (w410:i16)
    n329 = global read "系统设置全局变量.vi" "流量阈值"() -> (w408:dbl)
    n330 = global read "系统设置全局变量.vi" "时间阈值"() -> (w407:u16)
    n331 = global read "系统设置全局变量.vi" "运行模式"() -> (w409:enum16{"维护模式", "常规模式", "应急模式", "质控模式"})
    n332 = global read "系统设置全局变量.vi" "周期设置"() -> (w411:enum16{"自由设定", "国标协议", "流量设定"})
    n333 = global read "系统设置全局变量.vi" "氨氮自动启动设置"() -> (w423:bool)
    n334 = global read "系统设置全局变量.vi" "总磷自动启动设置"() -> (w406:bool)
    n335 = global read "系统设置全局变量.vi" "总氮自动启动设置"() -> (w421:bool)
    n336 = property class="VI"(reference=w418) -> (reference out=w415:refnum<vi>, "Exec.State"=w417:T6)  [unwired: 1 in, 1 out]
    n337 = Wait (ms)(milliseconds to wait=u32 1000 ("等待时间（毫秒）")) -> ()  [unwired: 1 out]
    n338 = global read "系统设置全局变量.vi" "质控启动日期"() -> (w414:string)
    n339 = global read "系统设置全局变量.vi" "24H周期设置"() -> (w424:bool[])
    n340 = global read "系统设置全局变量.vi" "跨度核查时间"() -> (w412:u16)
    n341 = global read "系统设置全局变量.vi" "空白核查时间"() -> (w413:u16)
    n342 = global read "系统设置全局变量.vi" "CODmn自动启动设置"() -> (w420:bool)
    n343 = global read "系统设置全局变量.vi" "CODCr自动启动设置"() -> (w422:bool)
    n344 = global read "系统设置全局变量.vi" "多参数自动启动设置"() -> (w419:bool)
    n345 = case shown="\"Idle\"" w417 {
      tunnel: w416 -> [_ w427 w435]
      tunnel: w415 -> [_ w428 w436]
      frame "Bad", Default {
      }
      frame "Idle" {
        n346 = case shown="假" w427 {
          tunnel: w428 -> [_ w434]
          frame False {
          }
          frame True {
            n347 = invoke class="VI" method="Run VI"(reference=w434, "Wait until done"=FALSE ("结束前等待"), "Auto Dispose Ref"=FALSE ("自动销毁引用")) -> (reference out=w429:refnum<vi>)  [unwired: 2 in, 4 out]
            n348 = invoke class="VI" method="FP.Open"(reference=w429, "Activate"=TRUE ("激活？"), "State"=T13."Standard" ("状态")) -> ()  [unwired: 2 in, 5 out]
          }
        }
      }
      frame "Run top level" {
        n349 = case shown="假" w435 {
          tunnel: w436 -> [w437 _]
          frame False {
            n350 = invoke class="VI" method="Abort VI"(reference=w437) -> (reference out=w438:refnum<vi>)  [unwired: 2 in, 2 out]
            n351 = invoke class="VI" method="FP.Close"(reference=w438) -> ()  [unwired: 2 in, 3 out]
          }
          frame True {
          }
        }
      }
    }
    n352 = local write "运行间隔"(w410) -> ()
    n353 = local write "流量阈值"(w408) -> ()
    n354 = local write "时间阈值"(w407) -> ()
    n355 = local write "运行模式"(w409) -> ()
    n356 = local write "周期设置"(w411) -> ()
    n357 = local write "质控启动日期"(w414) -> ()
    n358 = local write "24H周期设置"(w424) -> ()
    n359 = local write "跨度核查时间"(w412) -> ()
    n360 = local write "空白核查时间"(w413) -> ()
    n361 = local write "氨氮"(w423) -> ()
    n362 = local write "总磷"(w406) -> ()
    n363 = local write "总氮"(w421) -> ()
    n364 = local write "多参数"(w419) -> ()
    n365 = local write "CODCr"(w422) -> ()
    n366 = local write "CODmn"(w420) -> ()
  }
